vi "Read ID.vi"(11 "Channel Message in":refnum<class "Channel Message.lvclass">) -> (1 "id":u32)   [LabVIEW 2017, in "Channel Message.lvclass"]
doc: "When a message is written to the channel, it is assigned an ID that is unique for that channel. The message IDs increment serially."
uses:
  <vilib>/ChannelSupport/Channel Message/Channel Message.lvclass
  <vilib>/ChannelSupport/Channel Message/Channel Message.lvclass/Channel Message.ctl
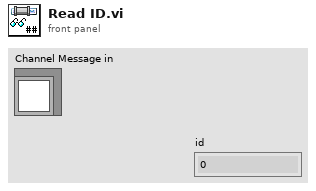
[diagram p1: front panel]
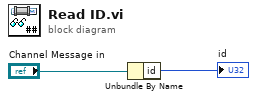
[diagram p0: block diagram]
diagram:
  n1 = Unbundle By Name("Channel Message in") -> ("id"=→"id":u32)
